vi "XNET Database Delete (Frame).vi"(0 "frame in":refnum<k21>, 11 "error in (no error)":errorcluster) -> (15 "error out":errorcluster)   [LabVIEW 2018]
doc: "Deletes a frame and all child objects in this frame."
uses:
  nixlvapi.dll
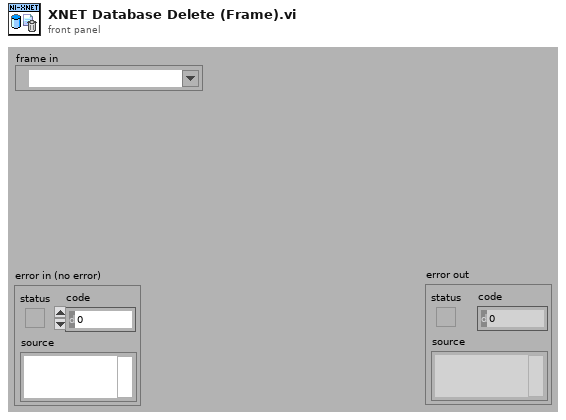
[diagram p1: front panel]
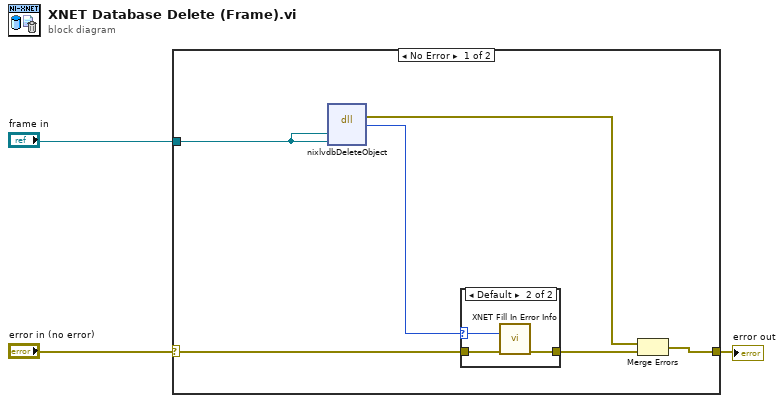
[diagram p0: block diagram]
diagram:
  n1 = case shown="No Error" "error in (no error)" {
    selector: "error in (no error)" -> [w8 w14]
    tunnel: "frame in" -> [w7 _]
    tunnel: [w5 w14] -> w3
    frame No Error {
      n2 = dll-call lib="nixlvapi.*" fn="nixlvdbDeleteObject" ("nilvxaiu.dll:lvxenDatabaseDeleteObject")("reference"=w7, "refObjPtr"=w7) -> (error out=w4:errorcluster, "return type"=w6:i32)  [unwired: 4 in, 2 out]
      n3 = case shown="Default" w6 {
        selector: w6 -> [_ w11]
        tunnel: w8 -> [w10 w12]
        tunnel: [w10 w13] -> w9
        frame 0 {
        }
        frame Default {
          n4 = call "XNET Fill In Error Info.vi"("status code"=w11, "error in"=w12) -> ("error out"=w13:errorcluster)  [unwired: 13 out]
        }
      }
      n5 = Merge Errors(w4, w9) -> (w5:errorcluster)
    }
    frame Error {
    }
  }
  "error out" <- w3
